vi "Solve1.vi"(8 "Error In":errorcluster, 11 "object in":refnum<class "2024_2.lvclass">) -> (0 "Error Out":errorcluster, 2 "Result":u64, 3 "object out":refnum<class "2024_2.lvclass">)   [LabVIEW 2023, in "2024_2.lvclass"]
uses:
  2024_2.lvclass
  2024_2.lvclass/2024_2.ctl
panel:
  out "Array":bool[](array[boolean])
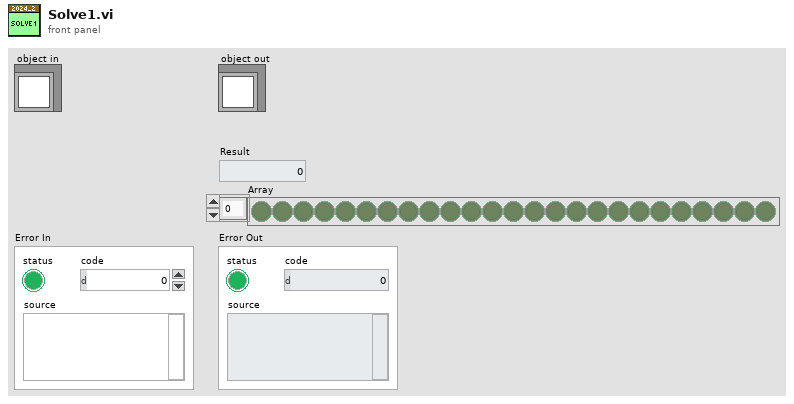
[diagram p1: front panel]
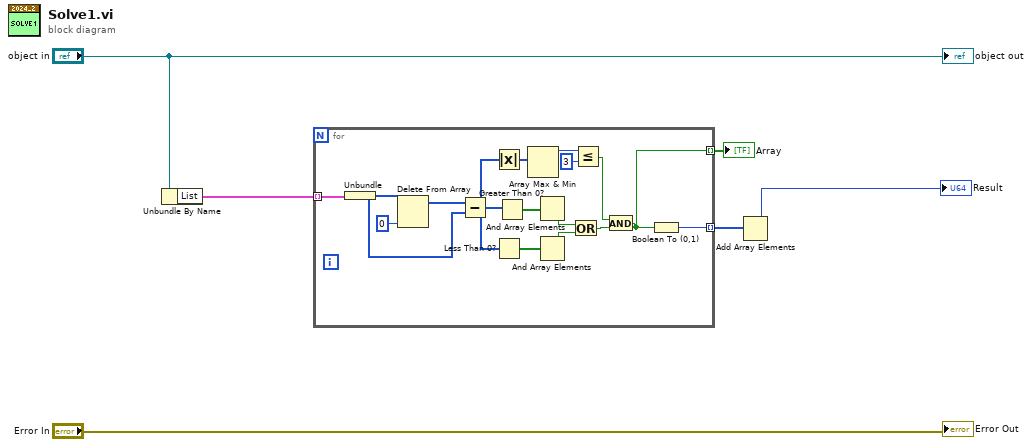
[diagram p0: block diagram]
diagram:
  n1 = Unbundle By Name("object in") -> ("List"=w4:cluster{"List":i32[]}[])
  n2 = for {
    tunnel: w4 -> [w22] mode=indexing
    tunnel: [w14] -> w3 mode=indexing
    tunnel: [w10] -> w1 mode=indexing
    n3 = Unbundle(w22) -> ("List"=w19:i32[])
    n4 = Delete From Array(array=w19, index=0) -> (array with subset deleted=w20:i32[])  [unwired: 1 in, 1 out]
    n5 = Subtract(x=w20, y=w19) -> (x-y=w12:i32[])
    n6 = Absolute Value(x=w12) -> (abs(x)=w11:i32[])
    n7 = Less Than 0?(x=w12) -> (x < 0?=w17:bool[])
    n8 = Greater Than 0?(x=w12) -> (x > 0?=w18:bool[])
    n9 = Array Max & Min(array=w11) -> (max value=w9:i32)  [unwired: 3 out]
    n10 = And Array Elements(Boolean array=w18) -> (logical AND=w16:bool)
    n11 = And Array Elements(Boolean array=w17) -> (logical AND=w15:bool)
    n12 = Or(x=w16, y=w15) -> (x .or. y?=w13:bool)
    n13 = Less Or Equal?(x=w9, y=3) -> (x <= y?=w8:bool)
    n14 = And(x=w8, y=w13) -> (x .and. y?=w10:bool)
    n15 = Boolean To (0,1)(Boolean=w10) -> (0, 1=w14:i16)
  }
  "Array" <- w1
  n16 = Add Array Elements(numeric array=w3) -> (sum=→"Result":i16)
  "Error Out" <- "Error In"
  "object out" <- "object in"
